vi "integracao_1.0.vi"() -> ()   [LabVIEW 2011]
panel:
  out "Integral":dbl
  out "pico real":bool
  out "slope negativo":bool
  out "slope positivo":bool
  out "delta tempo menor 0,025":bool
  out "sinal menor que 1":bool
  out "signal 2":dbl
  out "Boolean 3":bool
  out "tempo":dbl
  out "Boolean 2":bool
  out "Waveform Chart 2":dynamicdata(graph)
  out "Boolean":bool
  out "slop curve":dbl
  out "Result":dbl
  out "Waveform Chart":dynamicdata(graph)
  in  "Filename":path=path "C:/works/CG3000/datalog/gc3000_15-03-31_1222.lvm"
  out "signal":dbl
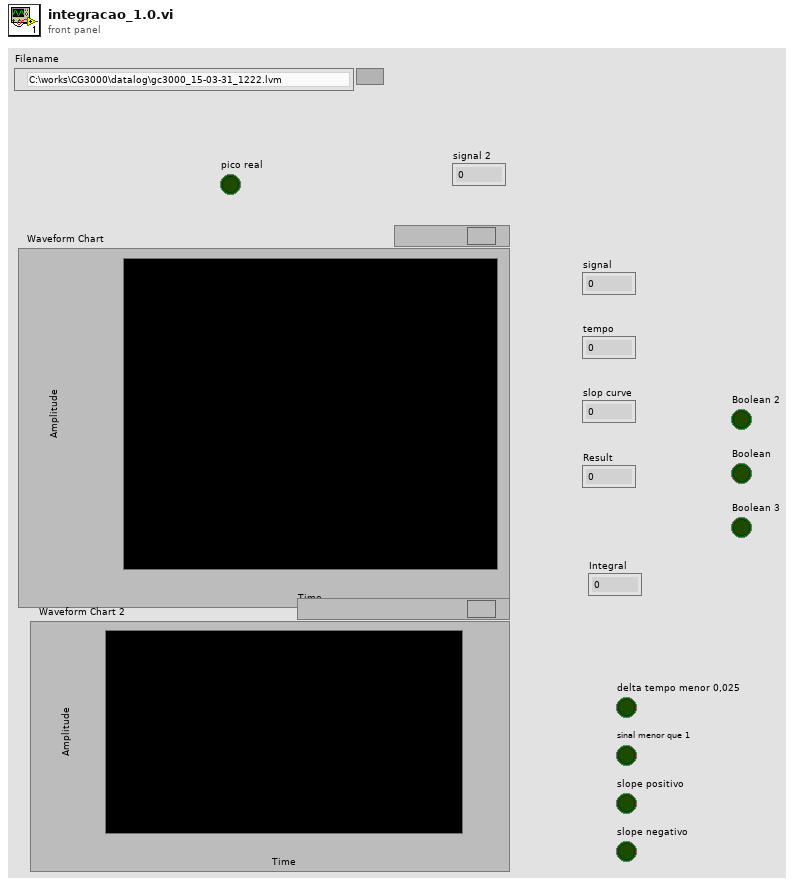
[diagram p1: front panel]
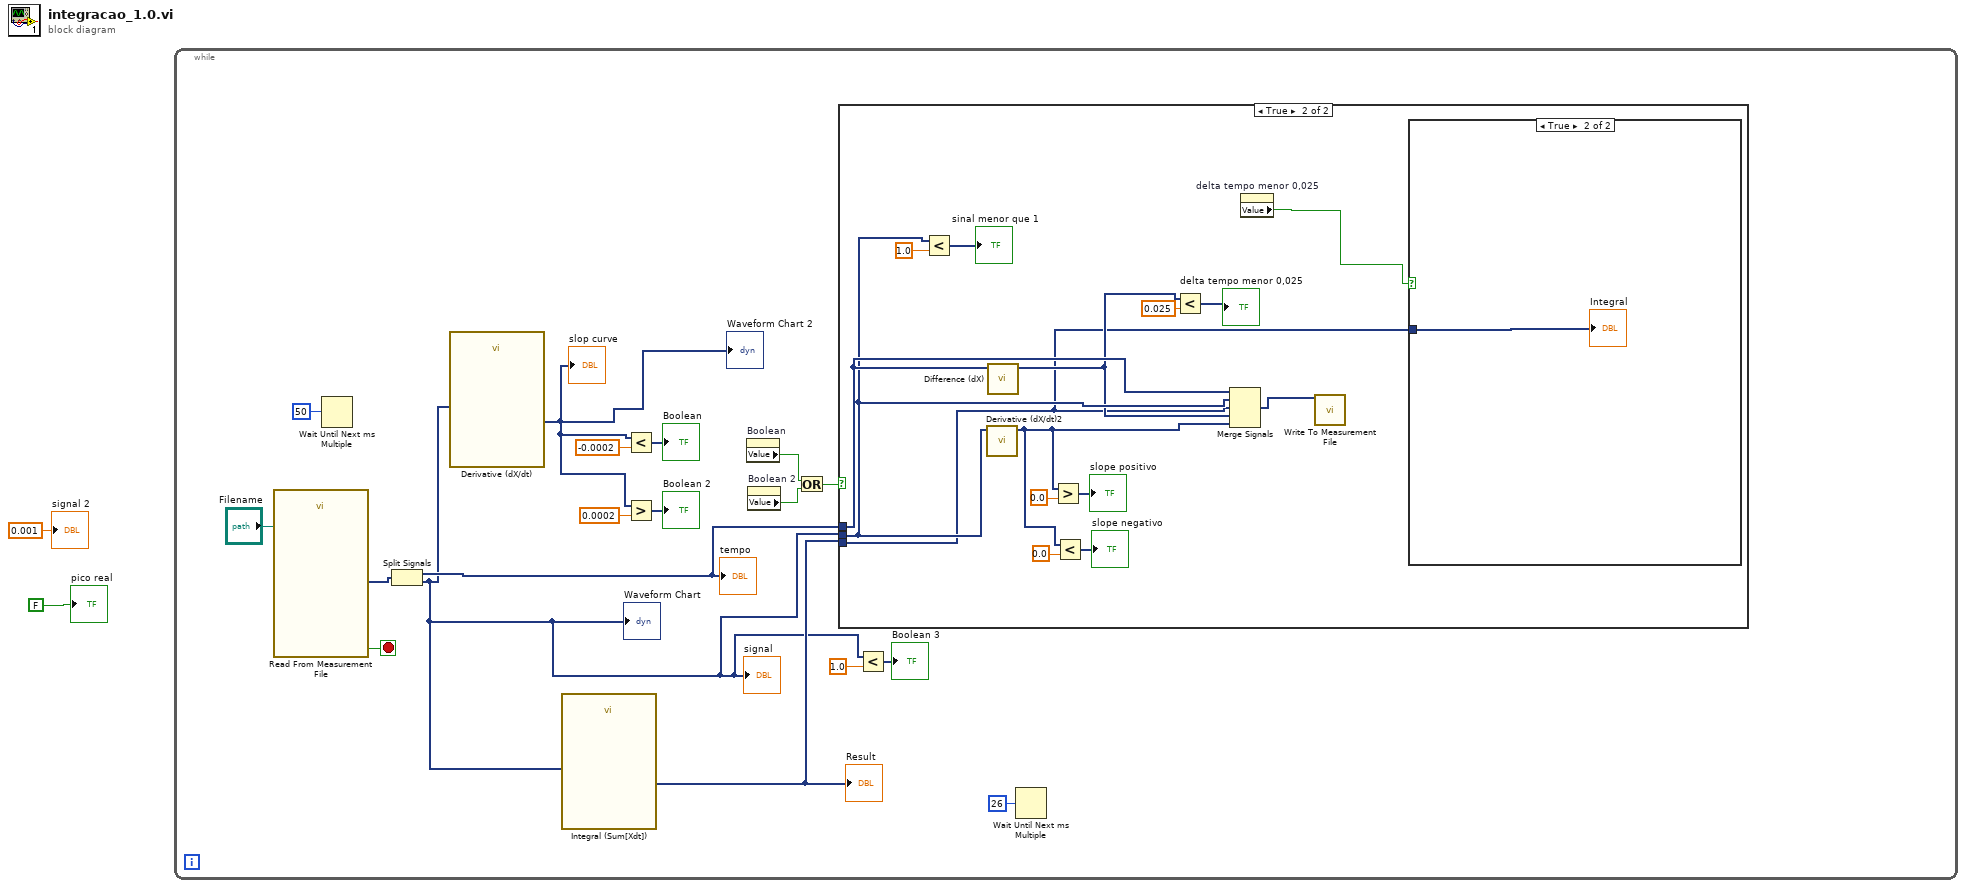
[diagram p0: block diagram]
diagram:
  n1 = while {
    stop <- w19 stop-if-true
    n2 = call "Read From Measurement File"("Filename"="Filename") -> ("Signals"=w13:dynamicdata, "EOF?"=w19:bool)  [unwired: 5 in, 4 out]
    n3 = Wait Until Next ms Multiple(millisecond multiple=u32 50) -> ()  [unwired: 1 out]
    n4 = Split Signals(w13) -> (w12:dynamicdata, w5:dynamicdata)  [unwired: 2 in]
    "signal" <- w5
    "Waveform Chart" <- w5
    "tempo" <- w12
    n5 = call "Derivative (dX/dt)"("Signals"=w5) -> ("Result"=w3:dynamicdata)  [unwired: 5 in, 1 out]
    "slop curve" <- w3
    "Waveform Chart 2" <- w3
    n6 = call "Integral (Sum[Xdt])"("Signals"=w5) -> ("Result"=w7:dynamicdata)  [unwired: 5 in, 1 out]
    "Result" <- w7
    n7 = Less?(x=w3, y=-0.0002) -> (x < y?=→"Boolean":dynamicdata)
    n8 = Greater?(x=w3, y=0.0002) -> (0:→"Boolean 2":dynamicdata)
    n9 = property on="Boolean" class="Bool (strict)"() -> ("Value"=w10:bool)  [unwired: 2 in, 2 out]
    n10 = property on="Boolean 2" class="Bool (strict)"() -> ("Value"=w9:bool)  [unwired: 2 in, 2 out]
    n11 = Or(x=w10, y=w9) -> (x .or. y?=w8:bool)
    n12 = case shown="True" w8 {
      tunnel: w12 -> [_ w34]
      tunnel: w5 -> [_ w33]
      tunnel: w7 -> [_ w21]
      frame False {
      }
      frame True {
        n13 = Less?(x=w33, y=1.0) -> (x < y?=→"sinal menor que 1":dynamicdata)
        n14 = call "Derivative (dX/dt)2"("Signals"=w33) -> ("Result"=w25:dynamicdata)  [unwired: 5 in, 1 out]
        n15 = call "Difference (dX)"("Signals"=w34) -> ("Result"=w30:dynamicdata)  [unwired: 5 in, 1 out]
        n16 = Greater?(x=w25, y=0.0) -> (0:→"slope positivo":dynamicdata)
        n17 = Less?(x=w25, y=0.0) -> (x < y?=→"slope negativo":dynamicdata)
        n18 = Less?(x=w30, y=0.025) -> (x < y?=→"delta tempo menor 0,025":dynamicdata)
        n19 = Merge Signals(w34, w33, w21, w30, w25) -> (w35:dynamicdata)
        n20 = property on="delta tempo menor 0,025" class="Bool (strict)"() -> ("Value"=w22:bool)  [unwired: 2 in, 2 out]
        n21 = call "Write To Measurement File"("Signals"=w35) -> ()  [unwired: 16 in, 3 out]
        n22 = case shown="True" w22 {
          tunnel: w21 -> [_ w36]
          frame False {
          }
          frame True {
            "Integral" <- w36
          }
        }
      }
    }
    n23 = Less?(x=w5, y=1.0) -> (x < y?=→"Boolean 3":dynamicdata)
    n24 = Wait Until Next ms Multiple(millisecond multiple=u32 26) -> ()  [unwired: 1 out]
  }
  "signal 2" <- 0.001 ("signal 2")
  "pico real" <- FALSE ("pico real")
